vi "PH_DeformableMirror.SetChannel.vi"(0 "i ref in":refnum<vi>, 1 "Channel":u32, 3 "Voltage":dbl, 4 "Hysteresis Compensation? (false)":bool, 5 "error in":errorcluster) -> (14 "i ref out":refnum<vi>, 19 "error out":errorcluster)   [LabVIEW 2014, in "PH_DeformableMirror.lvlib"]
uses:
  PH_DeformableMirror.lvlib
  instr.lib/dmdriver/DMirrorBase/DMirrorBase.lvclass
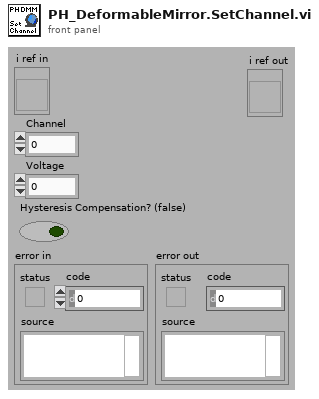
[diagram p1: front panel]
types:
  T1 = typedef "PH_DeformableMirror.lvlib/PH_DeformableMirror.i attribute.ctl" = cluster{"DMirror.lvlib:DMirrorBase.lvclass":refnum<class "DMirrorBase.lvclass">, "Device error":errorcluster, "GUI Refs":cluster{"Delete":refnum<vi>, "Device Error":refnum<vi>, "HV on":refnum<vi>, "Channel":refnum<vi>, "Voltage":refnum<vi>, "Channel Voltages":refnum<vi>}}
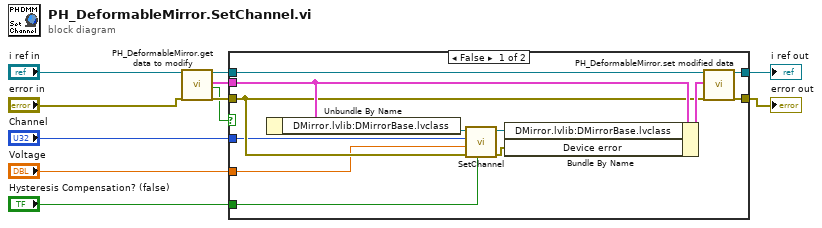
[diagram p0: block diagram]
diagram:
  n1 = call "PH_DeformableMirror.get data to modify.vi"("i ref in"="i ref in", "error in (no error)"="error in") -> ("i ref out"=w11:refnum<vi>, "i attribute"=w10:T1, "timed out"=w8:bool, "error out"=w9:errorcluster)  [unwired: 14 in]
  n2 = case shown="False" w8 {
    tunnel: [w23 w25] -> w6
    tunnel: w11 -> [w22 w25]
    tunnel: [w21 w24] -> w5
    tunnel: w9 -> [w15 w24]
    tunnel: w10 -> [w20 _]
    tunnel: "Channel" -> [w14 _]
    tunnel: "Voltage" -> [w13 _]
    tunnel: "Hysteresis Compensation? (false)" -> [w12 _]
    frame False {
      n3 = Unbundle By Name(w20) -> ("DMirror.lvlib:DMirrorBase.lvclass"=w19:refnum<class "DMirrorBase.lvclass">)
      n4 = call-dynamic "SetChannel.vi"("Hysteresis Compensation? (no)"=w12, "error in (no error)"=w15, "Voltage [V]"=w13, "Channel"=w14, "DMirrorBase in"=w19) -> ("error out"=w16:errorcluster, "DMirrorBase out"=w17:refnum<class "DMirrorBase.lvclass">)  [unwired: 5 in]
      n5 = Bundle By Name(cluster=w20, "DMirror.lvlib:DMirrorBase.lvclass"=w17, "Device error"=w16) -> (w18:T1)
      n6 = call "PH_DeformableMirror.set modified data.vi"("i ref in"=w22, "i attribute"=w18, "error in (no error)"=w15) -> ("i ref out"=w23:refnum<vi>, "error out"=w21:errorcluster)  [unwired: 15 in]
    }
    frame True {
    }
  }
  "error out" <- w5
  "i ref out" <- w6
